vi "openRemoteImage.vi"(8 "error in (no error)":errorcluster, 10 "remotePath":path, 11 "ImageStreamDecoder in":refnum<class "ImageStreamDecoder.lvclass">) -> (0 "error out":errorcluster, 2 "Image Out":T1, 3 "ImageStreamDecoder out":refnum<class "ImageStreamDecoder.lvclass">)   [LabVIEW 2009, in "Hardware.lvlib" / "HWControllers.lvlib" / "ImageStreamDecoder.lvclass"]
uses:
  ImageStreamDecoder.lvclass
  <vilib>/vision/Image Controls.llb/IMAQ Image.ctl
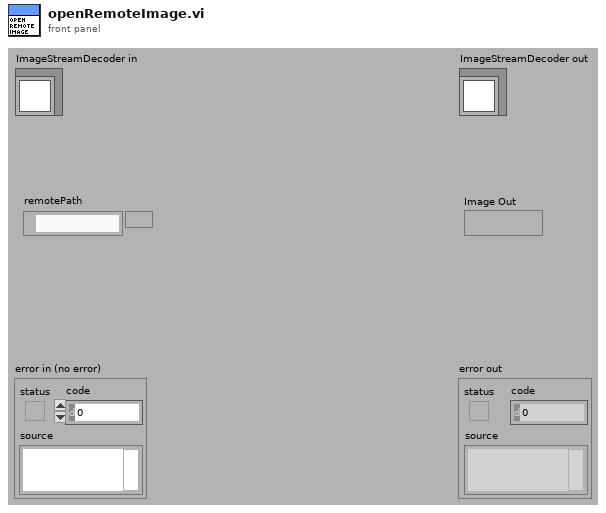
[diagram p1: front panel]
types:
  T1 = typedef "IMAQ Image.ctl" = refnum<image>
  T2 = typedef "Image Type" = u32
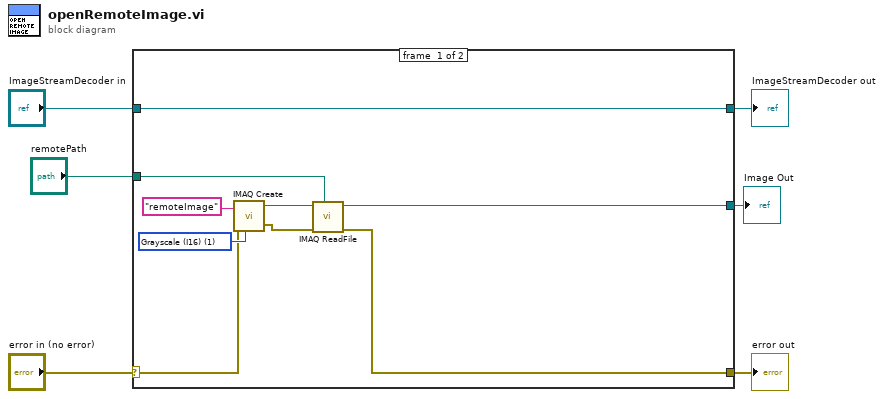
[diagram p0: block diagram]
diagram:
  n1 = case shown="No Error" "error in (no error)" {
    selector: "error in (no error)" -> [w9 w17]
    tunnel: [w8 w17] -> w5
    tunnel: [w15 w16] -> w3
    tunnel: "ImageStreamDecoder in" -> [w15 w16]
    tunnel: "remotePath" -> [w12 _]
    tunnel: [w7 _] -> w1
    frame #0 {
      w11 = T2 1 items=["Grayscale (U8)", "Grayscale (I16)", "Grayscale (SGL)", "Complex (CSG)", "RGB (U32)", "HSL (U32)", "RGB (U64)", "Grayscale (U16)"] ("Image Type")
      n2 = call "IMAQ Create"("Image Name"="remoteImage", "Image Type"=w11, "error in (no error)"=w9) -> ("New Image"=w14:T1, "error out"=w13:errorcluster)  [unwired: 2 in]
      n3 = call "IMAQ ReadFile"("File Path"=w12, "error in (no error)"=w13, "Image"=w14) -> ("error out"=w8:errorcluster, "Image Out"=w7:T1)  [unwired: 4 in, 3 out]
    }
    frame #1 {
    }
  }
  "error out" <- w5
  "ImageStreamDecoder out" <- w3
  "Image Out" <- w1
